vi "NumIntegrate_Rkdp_Mat_X_U.vi"(5 "Func_X_U_Extra":T1, 6 "MaxError":dbl=1e-06, 7 "PassedData":variant, 8 "dT_Seconds":dbl, 10 "U":T2, 11 "X":T2) -> (0 "Error":bool, 1 "IterationCount":i32, 3 "Return X":T2)   [LabVIEW 2019, in "Trajectory_Library.lvlib"]
doc: "Performs adaptive Dormand-Prince integration of dx/dt = f(x, u) for dt. By default, the max error is 1e-6.\n\n\n\nInputs:\n - Func_X_U_Extra -- A strictly typed LabVIEW reference to a function to integrate as a function of matrix X, U, and the extra passed data\n - PassedData -- This is a variant that can be used to pass additional data to the function if needed. The data must be packed into the variant in the specific way expected by the function.\n - X -- X input matrix\n - U -- U input matrix.\n - dT -- The time over which to integrate\n - maxError -- The maximum acceptable truncation error. Usually a small number like 1e-6.\n\nOutputs:\n - Return X -- the integration of dx/dt = f(x, u) for dt.\n - Error -- If TRUE, an error occured.\n - Iteration Count -- The number of times the integration iterated to reach the desired maxError."
uses:
  Trajectory_Library.lvlib
  <vilib>/Analysis/Matrix/Datatypes/RealMatrix.ctl
  CALLBACK_FUNC_TYPE.ctl
  NumIntegrate_Rkdp_Func_A.vi
  NumIntegrate_Rkdp_Func_B1B2.vi
  Matrix_NormF.vi
  NumIntegrate_Rkdp_Func_B1.vi
  NumIntegrate_Rkdp_Func_B2.vi
  <vilib>/Analysis/_algsub.llb/Matrix Norm.vi
  <vilib>/Analysis/_algsub.llb/Real Matrix Norm.vi
  <vilib>/Analysis/Matrix/Numeric/Multiply/Multiply.vi
  <vilib>/Analysis/Matrix/Numeric/Multiply/Multiply - RM,R.vi
  <vilib>/Analysis/Matrix/Numeric/Add/Add.vi
  <vilib>/Analysis/Matrix/Numeric/Add/Add - RM,RM.vi
  <vilib>/Analysis/Matrix/NI_Matrix.lvlib
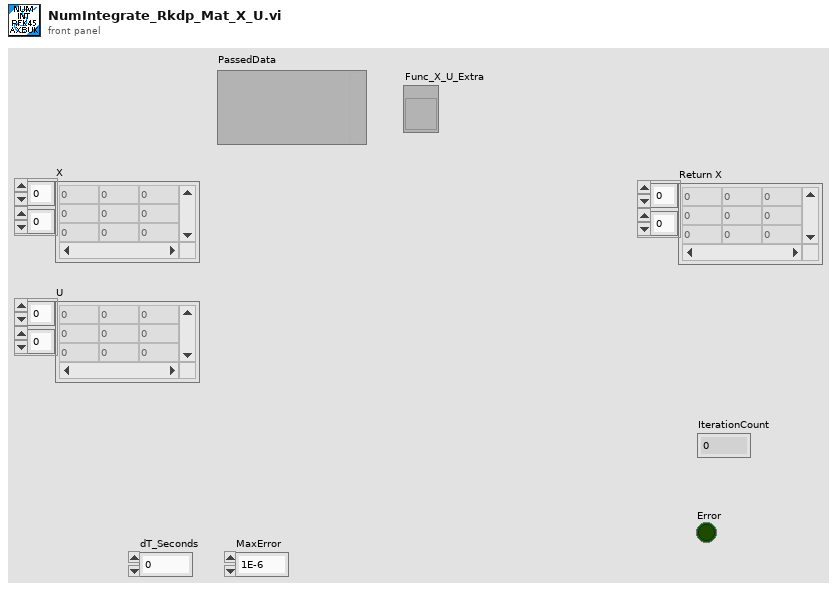
[diagram p1: front panel]
types:
  T1 = typedef "Trajectory_Library.lvlib/CALLBACK_FUNC_TYPE.ctl" = refnum<vi>
  T2 = typedef "NI_Matrix.lvlib/RealMatrix.ctl" = dbl[][]
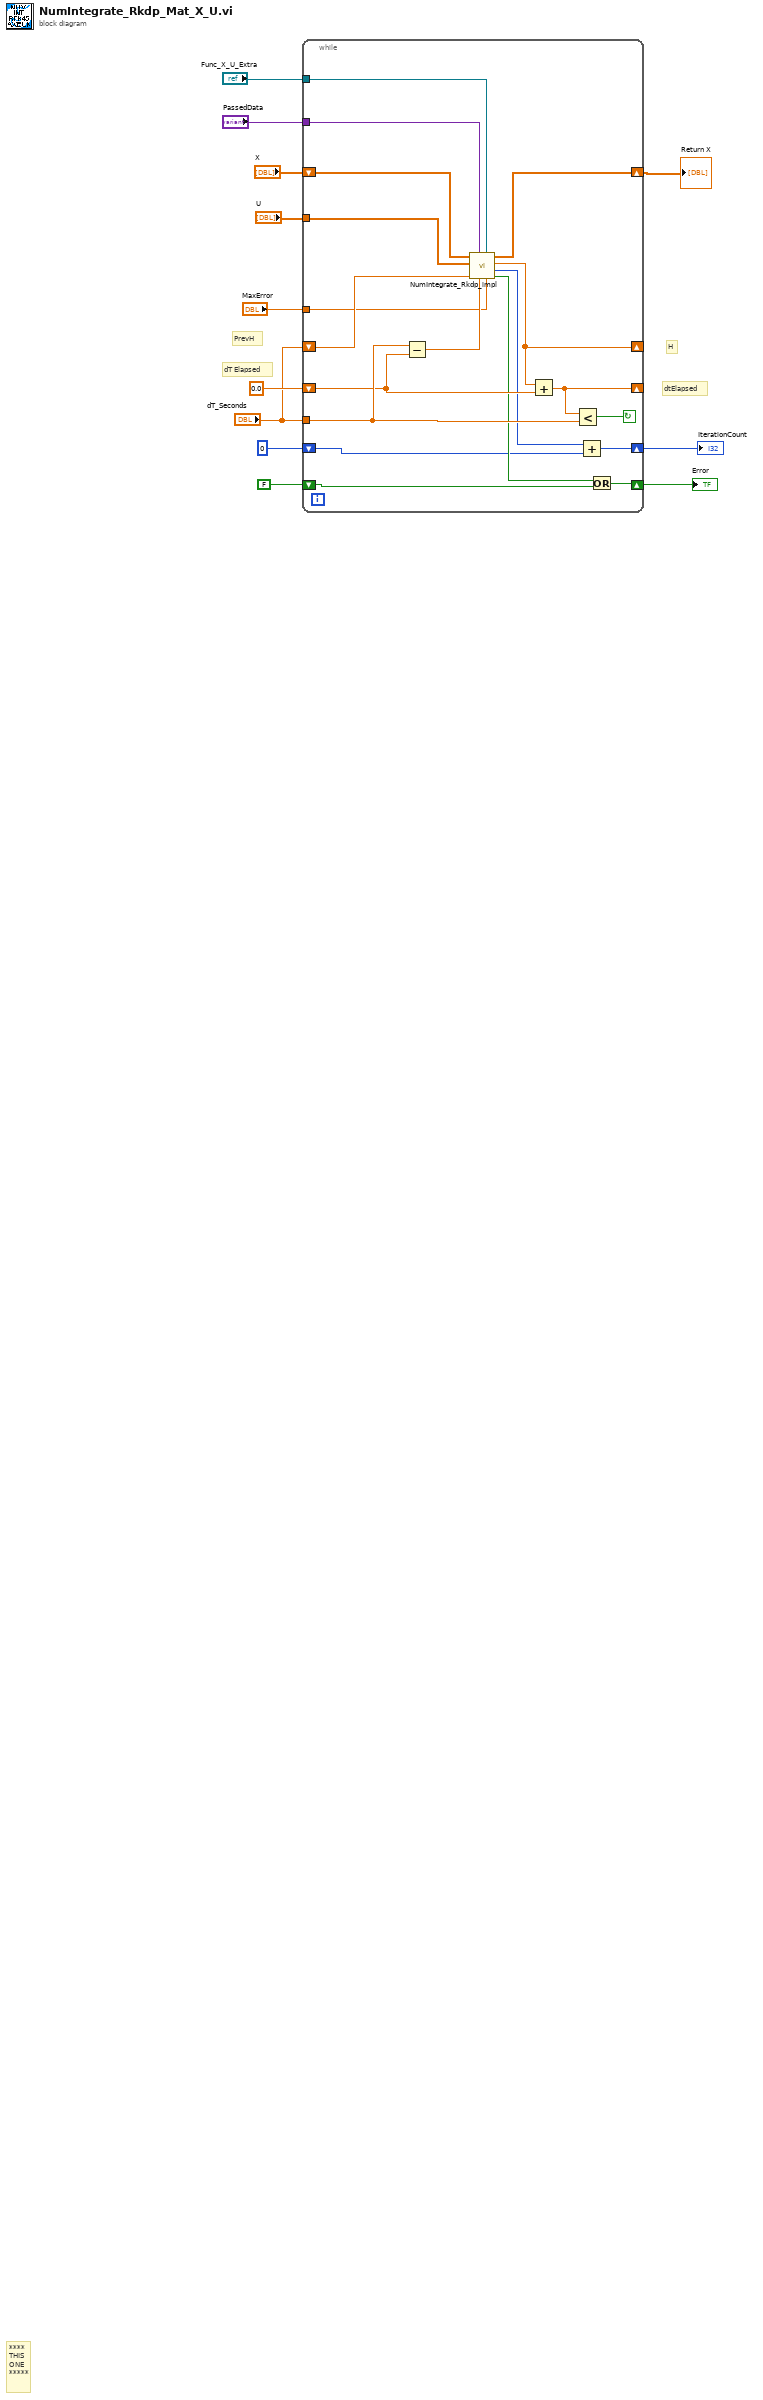
[diagram p0: block diagram]
diagram:
  # "H"
  # "dtElapsed"
  # "PrevH"
  # "dT Elapsed"
  # "****\nTHIS\nONE\n*****"
  n1 = while {
    shift-right: [w23] -> _
    shift-left: 0.0 -> [w22]
    tunnel: "dT_Seconds" -> [w26]
    shift-right: [w21] -> _
    shift-left: "dT_Seconds" -> [w27]
    shift-right: [w29] -> w8
    shift-left: "X" -> [w30]
    tunnel: "U" -> [w28]
    tunnel: "MaxError" -> [w24]
    tunnel: "Func_X_U_Extra" -> [w20]
    tunnel: "PassedData" -> [w19]
    shift-right: [w18] -> w3
    shift-left: FALSE -> [w17]
    shift-right: [w13] -> w1
    shift-left: 0 -> [w15]
    stop <- w31 continue-if-true
    n2 = Subtract(x=w26, y=w22) -> (x-y=w25:dbl)
    n3 = call "NumIntegrate_Rkdp_impl.vi"("MaxTruncError"=w24, "Func_X_U_Extra"=w20, "dT_Remaining"=w25, "PassedData"=w19, "InitialH"=w27, "U"=w28, "X"=w30) -> ("Error"=w16:bool, "IterationCount"=w14:i32, "H"=w21:dbl, "NewX"=w29:T2)  [unwired: 1 in]
    n4 = Add(x=w21, y=w22) -> (x+y=w23:dbl)
    n5 = Less?(x=w23, y=w26) -> (x < y?=w31:bool)
    n6 = Add(x=w14, y=w15) -> (x+y=w13:i32)
    n7 = Or(x=w16, y=w17) -> (x .or. y?=w18:bool)
  }
  "Return X" <- w8
  "IterationCount" <- w1
  "Error" <- w3
